vi "Cross Correlation Function.vi"(4 "Eng Values 2":dbl[](array[numeric]), 7 "Eng Values 1":dbl[](array[numeric])) -> (0 "error":i32, 1 "Delay index":i32, 2 "Max Cross Correlation":dbl, 3 "Cross Correlation":dbl[](array[numeric]))   [LabVIEW 2022 SP3]
uses:
  <vilib>/Analysis/2dsp.llb/1D Cross Correlation (DBL).vi
  <vilib>/Analysis/NI_AALPro.lvlib
  <vilib>/Analysis/NI_AALBase.lvlib
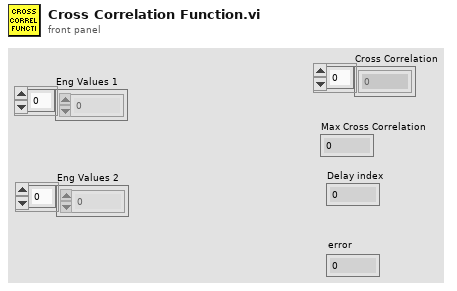
[diagram p1: front panel]
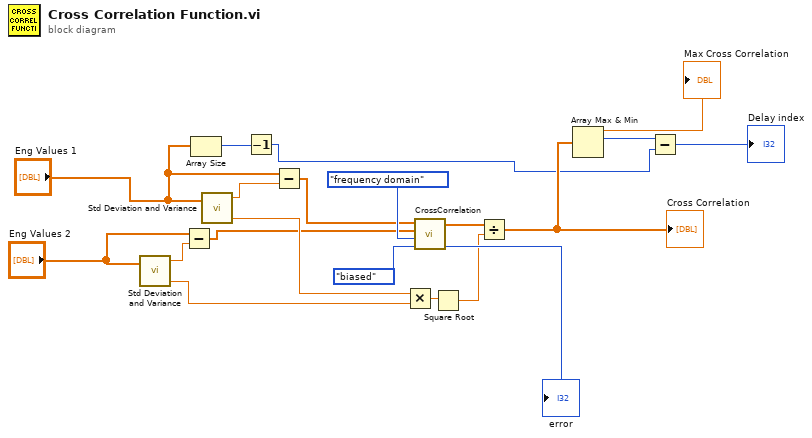
[diagram p0: block diagram]
diagram:
  n1 = call <vilib>:"Std Deviation and Variance.vi"("X"="Eng Values 2") -> ("mean"=w20:dbl, "variance"=w15:dbl)  [unwired: 1 in, 1 out]
  n2 = Subtract(x="Eng Values 2", y=w20) -> (x-y=w10:dbl[])
  n3 = Array Size(array="Eng Values 1") -> (size(s)=w6:i32)
  n4 = call <vilib>:"Std Deviation and Variance.vi"("X"="Eng Values 1") -> ("mean"=w19:dbl, "variance"=w16:dbl)  [unwired: 1 in, 1 out]
  n5 = Decrement(x=w6) -> (x-1=w3:i32)
  n6 = Subtract(x="Eng Values 1", y=w19) -> (x-y=w11:dbl[])
  n7 = Multiply(x=w16, y=w15) -> (x*y=w17:dbl)
  n8 = call-poly <vilib>:"CrossCorrelation.vi"("normalization"=enum32{"none", "unbiased", "biased"}."biased", "algorithm"=enum32{"direct", "frequency domain"}."frequency domain", "Y"=w10, "X"=w11) -> ("error"=→"error":i32, "Rxy"=w9:dbl[])  [unwired: 6 in]
  n9 = Square Root(x=w17) -> (sqrt(x)=w8:dbl)
  n10 = Divide(x=w9, y=w8) -> (x/y=w5:dbl[])
  "Cross Correlation" <- w5
  n11 = Array Max & Min(array=w5) -> (max value=→"Max Cross Correlation":dbl, max index (indices)=w4:i32)  [unwired: 2 out]
  n12 = Subtract(x=w4, y=w3) -> (x-y=→"Delay index":i32)
